vi "RefNums_Actuators.vi"() -> ()   [LabVIEW 2018]
panel:
  out "ButterflyPneumatic":string="FrontLeftDrive"
  out "Compressor":string="FrontLeftDrive"
  out "RobotDrive":string="FrontLeftDrive"
  out "FrontRightDrive":string="FrontLeftDrive"
  out "FrontLeftDrive":string="FrontLeftDrive"
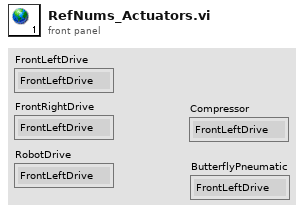
[diagram p1: front panel]
diagram:
